vi "myPICO_CheckNum.vi"(6 "需要的示波器台数":u8, 7 "当前log":string, 8 "最大检测设备数":i16=2, 9 "最大同时扫频数":u32=5 min=1 max=20, 10 "注入(1号)端口类型":u8(ring) items=["单相", "三相αβ系", "三相同步系", "三相正负序"], 11 "错误常量":errorcluster) -> (0 "可以正常测量":bool, 1 "实际驱动设备数":u16, 2 "序列号组 2":i8[][](array[numeric]), 3 "错误输出":errorcluster, 5 "更新log":string)   [LabVIEW 2024]
doc: "调用了库函数EnumerateUnits。\n根据需要的设备数，\n如果检测到的设备数不够，输出不可扫频的判断结果；\n如果足够或过多，输出扫频中实际需要用到大小的序列号二维数组，其中每行对应一台设备。\n同时，更新输出log。"
uses:
  ps2000a.dll
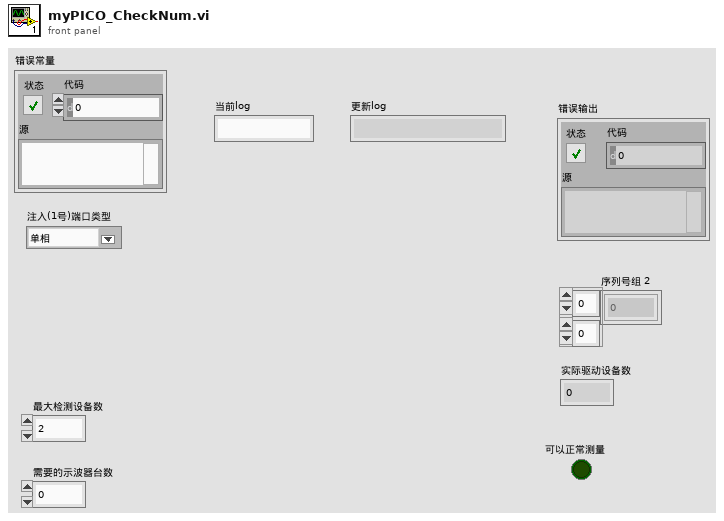
[diagram p1: front panel]
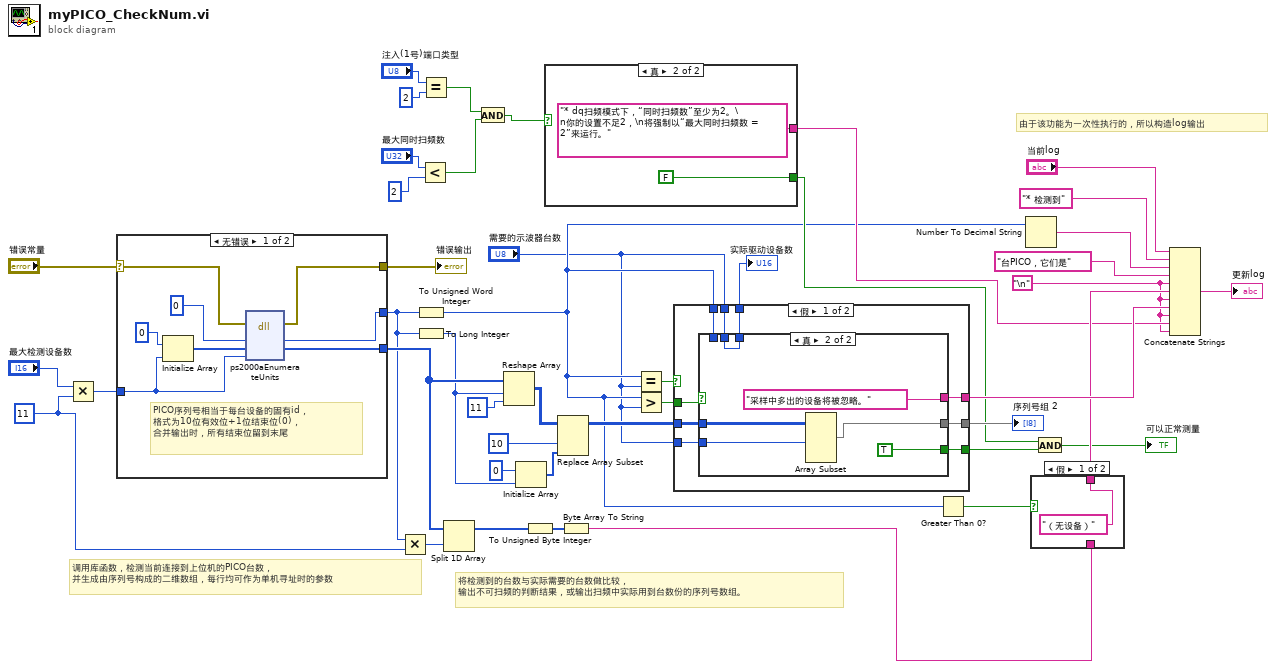
[diagram p0: block diagram]
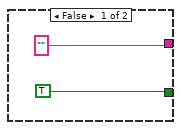
[diagram p3: hidden frame]
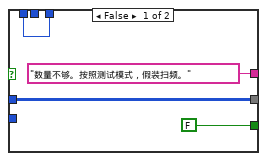
[diagram p4: hidden frame]
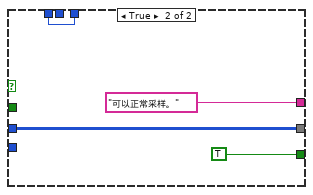
[diagram p5: hidden frame]
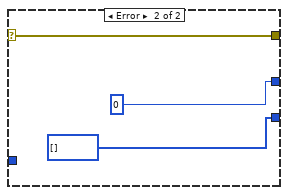
[diagram p6: hidden frame]
diagram:
  w4 = "\n"
  w31 = i16 11 ("new element/subarray")
  # "由于该功能为一次性执行的，所以构造log输出"
  # "将检测到的台数与实际需要的台数做比较，\n输出不可扫频的判断结果，或输出扫频中实际用到台数份的序列号数组。"
  # "调用库函数，检测当前连接到上位机的PICO台数，\n并生成由序列号构成的二维数组，每行均可作为单机寻址时的参数"
  n1 = Multiply(x="最大检测设备数", y=w31) -> (x*y=w35:i16)
  n2 = case shown="无错误" "错误常量" {
    selector: "错误常量" -> [w52 w55]
    tunnel: [w51 w55] -> w43
    tunnel: [w49 i16 0 ("count 2")] -> w19
    tunnel: [w48 i8[] [] ("serials 2")] -> w34
    tunnel: w35 -> [w45 _]
    frame No Error {
      # "PICO序列号相当于每台设备的固有id，\n格式为10位有效位+1位结束位(0)，\n合并输出时，所有结束位留到末尾"
      n3 = Initialize Array(i8 0 ("new element/subarray"), w45) -> (w46:i8[])
      n4 = dll-call lib="ps2000a.dll" fn="ps2000aEnumerateUnits"(error in=w52, "count"=i16 0, "serials"=w46, "serialLth"=w45) -> (error out=w51:errorcluster, "count"=w49:i16, "serials"=w48:i8[])  [unwired: 4 in, 1 out]
    }
    frame Error {
    }
  }
  "错误输出" <- w43
  n5 = Multiply(x=w19, y=w31) -> (x*y=w32:i16)
  n6 = To Unsigned Word Integer(number=w19) -> (unsigned 16bit integer=w2:u16)
  n7 = To Long Integer(number=w19) -> (32bit integer=w20:i32)
  n8 = Less?(x="最大同时扫频数", y=u32 2) -> (x < y?=w16:bool)
  n9 = Equal?(x="注入(1号)端口类型", y=u8 2) -> (x = y?=w12:bool)
  n10 = Split 1D Array(array=w34, index=w32) -> (first subarray=w33:i8[])  [unwired: 1 out]
  n11 = And(x=w12, y=w16) -> (x .and. y?=w15:bool)
  n12 = Reshape Array(w34, w20, 11 ("new element/subarray")) -> (w40:i8[][])
  n13 = Initialize Array(i8 0, w20) -> (w37:i8[])
  n14 = To Unsigned Byte Integer(number=w33) -> (unsigned 8bit integer=w36:u8[])
  n15 = case shown="真" w15 {
    tunnel: ["" "* dq扫频模式下，“同时扫频数”至少为2。\n你的设置不足2，\n将强制以“最大同时扫频数 = 2”来运行。"] -> w5
    tunnel: [TRUE FALSE] -> w8
    frame False {
    }
    frame True {
    }
  }
  n16 = Replace Array Subset(array=w40, new element=w37, index (col)=10 ("new element/subarray")) -> (w22:i8[][])  [unwired: 1 in]
  n17 = Byte Array To String(unsigned byte array=w36) -> (string=w10:string)
  n18 = Equal?(x=w2, y="需要的示波器台数") -> (x = y?=w27:bool)
  n19 = Greater?(x=w2, y="需要的示波器台数") -> (0:w26:bool)
  n20 = case shown="假" w27 {
    tunnel: w26 -> [w68 _]
    tunnel: [w67 "可以正常采样。"] -> w21
    tunnel: w22 -> [w66 w81]
    tunnel: [w65 w81] -> w25
    tunnel: "需要的示波器台数" -> [w64 _]
    tunnel: [w63 TRUE] -> w7
    tunnel: [w61 w79] -> w3
    tunnel: w2 -> [w62 w79]
    tunnel: "需要的示波器台数" -> [w60 _]
    frame False {
      n21 = case shown="真" w68 {
        tunnel: ["数量不够。按照测试模式，假装扫频。" "采样中多出的设备将被忽略。"] -> w67
        tunnel: w66 -> [w71 w77]
        tunnel: [w71 w76] -> w65
        tunnel: w64 -> [_ w75]
        tunnel: [FALSE TRUE] -> w63
        tunnel: w62 -> [w69 _]
        tunnel: [w69 w73] -> w61
        tunnel: w60 -> [_ w73]
        frame False {
        }
        frame True {
          n22 = Array Subset(array=w77, length (row)=w75) -> (w76:i8[][])  [unwired: 3 in]
        }
      }
    }
    frame True {
    }
  }
  "序列号组 2" <- w25
  "实际驱动设备数" <- w3
  n23 = Greater Than 0?(x=w2) -> (x > 0?=w11:bool)
  n24 = Number To Decimal String(number=w2) -> (decimal integer string=w30:string)  [unwired: 1 in]
  n25 = case shown="假" w11 {
    tunnel: w10 -> [_ w84]
    tunnel: ["（无设备）" w84] -> w9
    frame False {
    }
    frame True {
    }
  }
  n26 = And(x=w8, y=w7) -> (x .and. y?=→"可以正常测量":bool)
  n27 = Concatenate Strings("当前log", "* 检测到", w30, "台PICO，它们是", w4, w9, w4, w21, w4, w5, w4) -> (→"更新log":string)
